vi "Adapt and Append Waveform.vi"(8 "Error":errorcluster, 9 "Raw Waveform":T1, 11 "WavBuf":refnum<class "(WavBuf).lvclass">) -> (0 "Error Out":errorcluster, 3 "WavBuf Out":refnum<class "(WavBuf).lvclass">)   [LabVIEW 2016, in "(WavBuf).lvclass"]
uses:
  (WavBuf).lvclass
  Universal Controls/Waveform_Data.ctl
  (WavBuf).lvclass/(WavBuf).ctl
  Support/Waveform_Append and Resize Allocated.vi
  Support/Waveform_Read Write End Point Index.vi
  <vilib>/Waveform/WDTOps.llb/Get Final Time Value.vi
  <vilib>/Waveform/WDTOps.llb/WDT Get Final Time Value DBL.vi
  Support/PointerArray_Offset.vi
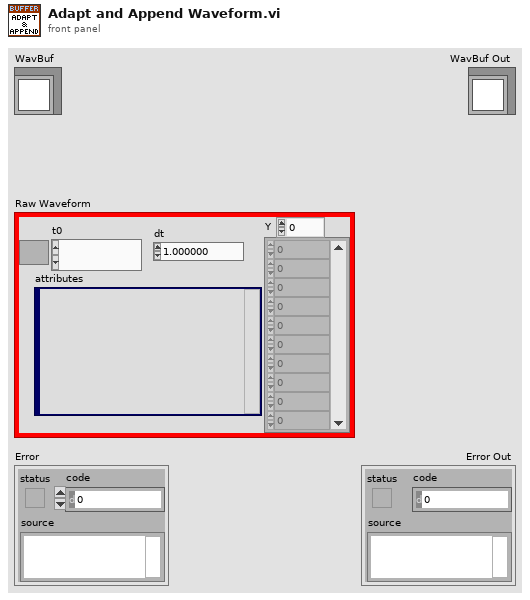
[diagram p1: front panel]
types:
  T1 = typedef "Waveform_Data.ctl" = waveform(dbl)
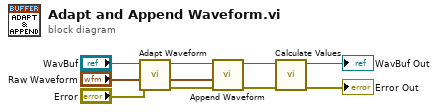
[diagram p0: block diagram]
diagram:
  n1 = call-dynamic "Adapt Waveform.vi"("Error"="Error", "Waveform"="Raw Waveform", "(WavBuf)"="WavBuf") -> ("Error Out"=w2:errorcluster, "Waveform Out"=w3:T1, "(WavBuf) Out"=w5:refnum<class "(WavBuf).lvclass">)  [unwired: 6 in]
  n2 = call "Append Waveform.vi"("Error"=w2, "Waveform To Append"=w3, "(WavBuf)"=w5) -> ("Error Out"=w1:errorcluster, "(WavBuf) Out"=w4:refnum<class "(WavBuf).lvclass">)  [unwired: 7 in]
  n3 = call-dynamic "Calculate Values.vi"("Error"=w1, "WavBuf"=w4) -> ("Error Out"=→"Error Out":errorcluster, "WavBuf Out"=→"WavBuf Out":refnum<class "(WavBuf).lvclass">)  [unwired: 8 in]
